vi "BreakupString.vi"(1 "bite size":i32=90000, 2 "data string":string) -> (0 "Array":string[](array[string]))   [LabVIEW 2018]
panel:
  out "Array 2":i32[](array[numeric])
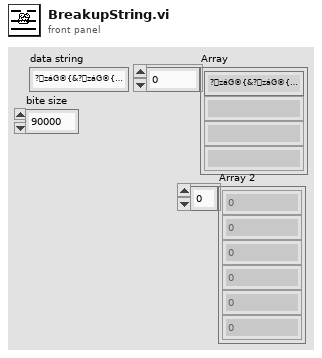
[diagram p1: front panel]
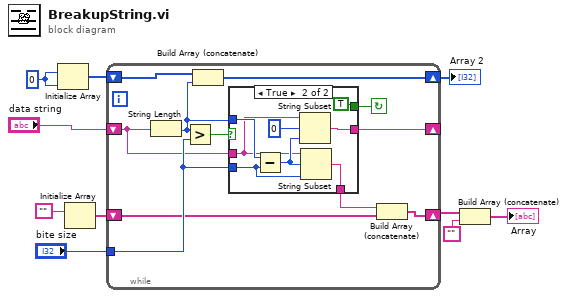
[diagram p0: block diagram]
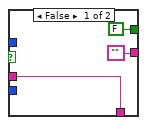
[diagram p2: hidden frame]
diagram:
  w2 = 0 ("bite size")
  n1 = Initialize Array(w2, w2) -> (w3:i32[])
  n2 = Initialize Array("") -> (w9:string[])  [unwired: 1 in]
  n3 = while {
    shift-right: [w21] -> _
    shift-left: "data string" -> [w14]
    shift-right: [w20] -> w5
    shift-left: w9 -> [w15]
    tunnel: "bite size" -> [w19]
    shift-right: [w12] -> w1
    shift-left: w3 -> [w11]
    stop <- w17 continue-if-true
    n4 = String Length(string=w14) -> (length=w13:i32)
    n5 = Greater?(x=w13, y=w19) -> (0:w18:bool)
    n6 = Build Array (concatenate)(w11, w13) -> (w12:i32[])
    n7 = case shown="True" w18 {
      tunnel: w13 -> [_ w32]
      tunnel: ["" w29] -> w21
      tunnel: [w24 w28] -> w16
      tunnel: w19 -> [_ w27]
      tunnel: w14 -> [w24 w26]
      tunnel: [FALSE TRUE] -> w17
      frame False {
      }
      frame True {
        n8 = Subtract(x=w32, y=w27) -> (x-y=w31:i32)
        n9 = String Subset(string=w26, offset (0)=0, length (rest)=w31) -> (substring=w29:string)
        n10 = String Subset(string=w26, offset (0)=w31, length (rest)=w27) -> (substring=w28:string)
      }
    }
    n11 = Build Array (concatenate)(w16, w15) -> (w20:string[])
  }
  "Array 2" <- w1
  n12 = Build Array (concatenate)(w5, "") -> (→"Array":string[])
